vi "Send Configurations To TestStand.vi"(8 "error in (no error)":errorcluster, 11 "TS UI Data in":T1) -> (0 "error out":errorcluster, 3 "TS UI Data out":T1)   [LabVIEW 2015]
uses:
  Type defs/TS UI Data.ctl
  Type defs/Variant Data Cluster.ctl
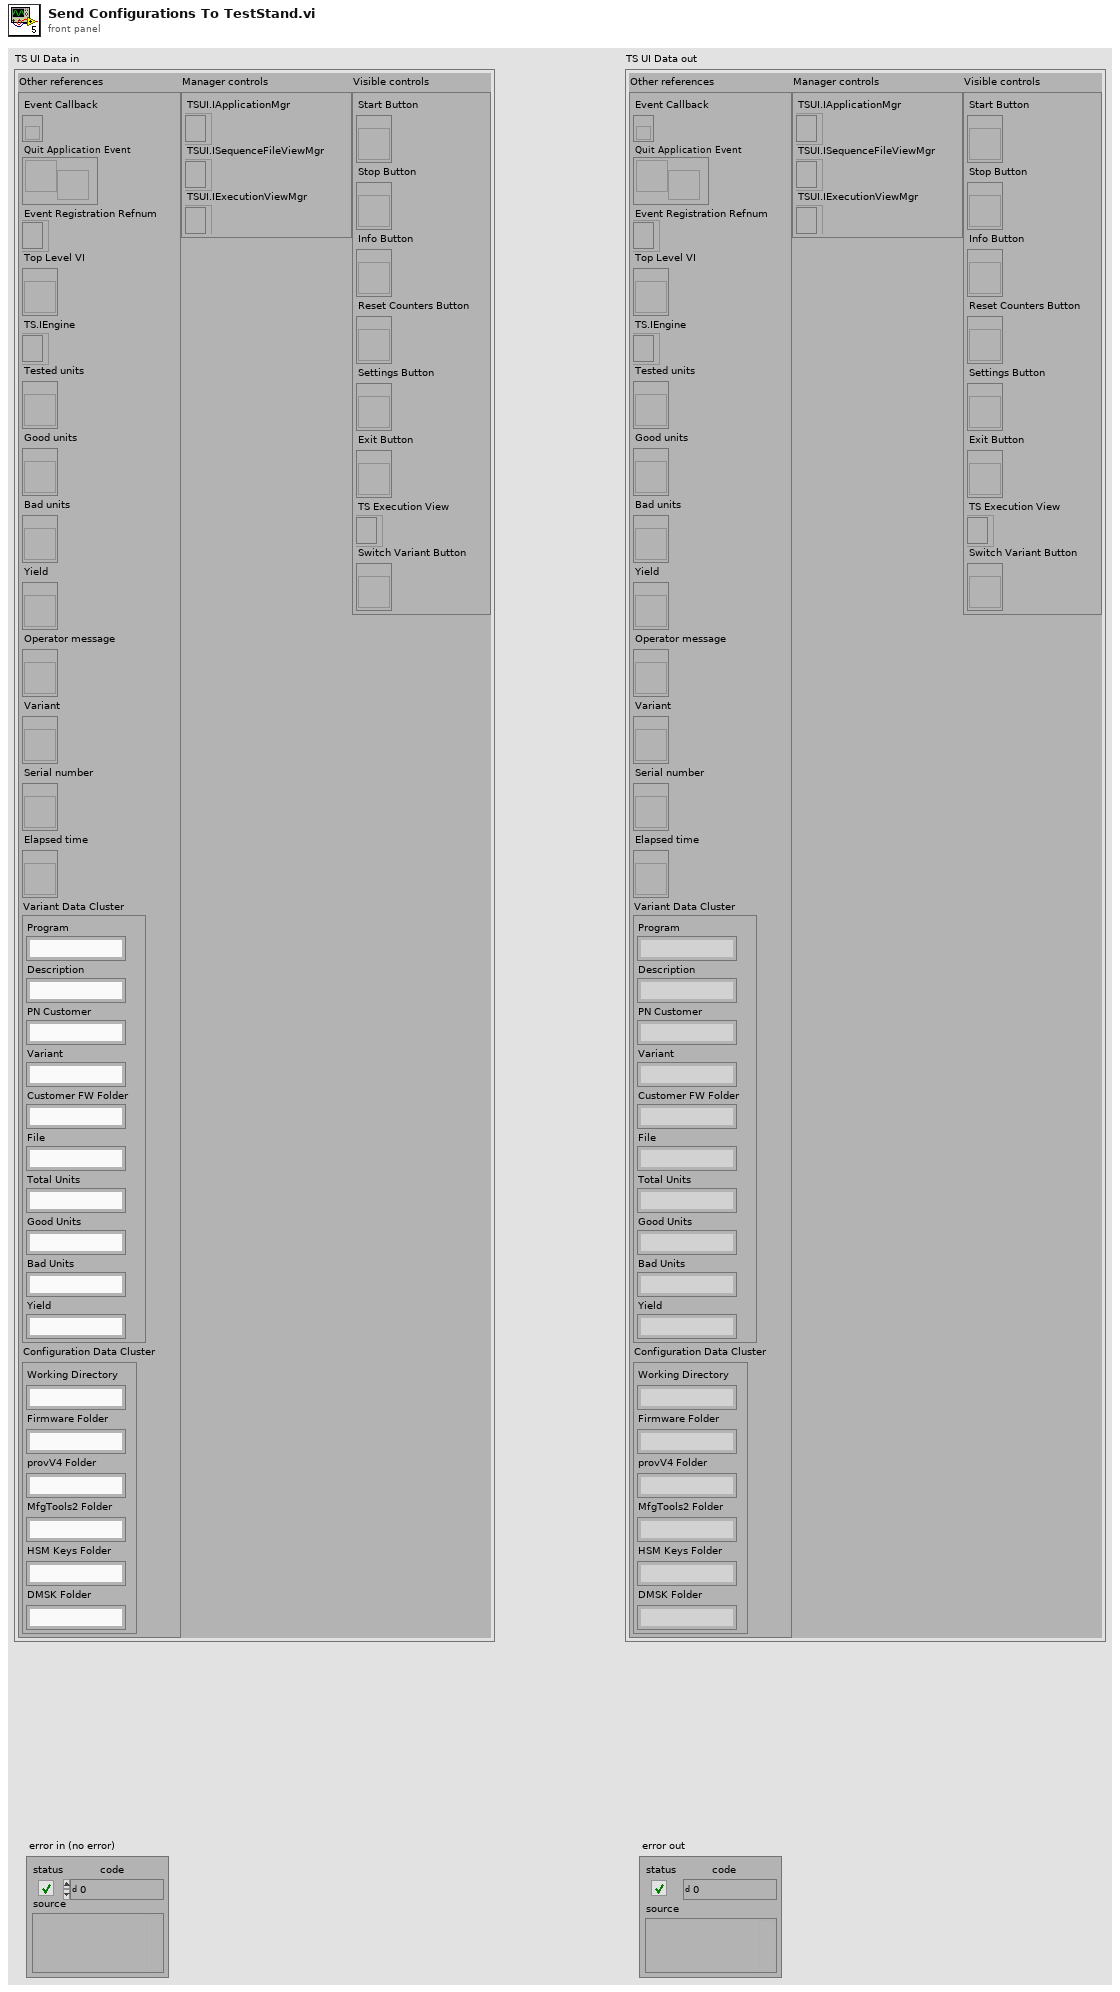
[diagram p1: front panel]
types:
  T1 = typedef "TS UI Data.ctl" = cluster{"Other references":cluster{"Event Callback":refnum<k27>, "Quit Application Event":refnum<user-event>, "event registration refnum":refnum<event-registration>, "Top Level VI":refnum<vi>, "TS.IEngine":refnum<k7>, "Tested units":refnum<vi>, "Good units":refnum<vi>, "Bad units":refnum<vi>, "Yield":refnum<vi>, "Operator message":refnum<vi>, "Variant":refnum<vi>, "Serial number":refnum<vi>, "Elapsed time":refnum<vi>, "Variant Data Cluster":T2, "Configuration Data Cluster":cluster{"Working Directory":string, "Firmware Folder":string, "provV4 Folder":string, "MfgTools2 Folder":string, "HSM Keys Folder":string, "DMSK Folder":string}}, "Manager controls":cluster{"TSUI.IApplicationMgr":refnum<k7>, "TSUI.ISequenceFileViewMgr":refnum<k7>, "TSUI.IExecutionViewMgr":refnum<k7>}, "Visible controls":cluster{"Start Button":refnum<vi>, "Stop Button":refnum<vi>, "Info Button":refnum<vi>, "Reset Counters Button":refnum<vi>, "Settings Button":refnum<vi>, "Exit Button":refnum<vi>, "TS Execution View":refnum<k7>, "Switch Variant Button":refnum<vi>}}
  T2 = typedef "Variant Data Cluster.ctl" = cluster{"Program":string, "Description":string, "PN Customer":string, "Variant":string, "Customer FW Folder":string, "File":string, "Total Units":string, "Good Units":string, "Bad Units":string, "Yield":string}
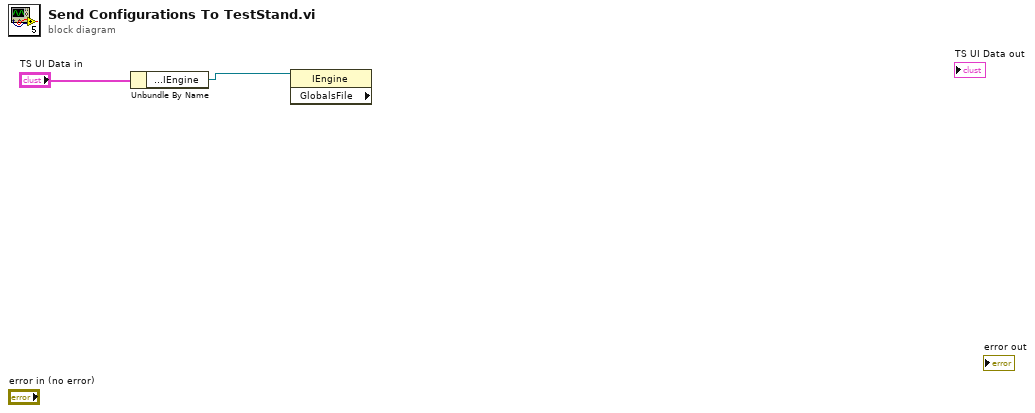
[diagram p0: block diagram]
diagram:
  n1 = Unbundle By Name("TS UI Data in") -> ("Other references.TS.IEngine"=w1:refnum<k7>)
  n2 = property class="IEngine" props=["GlobalsFile"](reference=w1) -> ()  [unwired: 1 in, 3 out]
